vi "Hand_Store_rach.vi"() -> ()   [LabVIEW 2016]
doc: "自动采集图线程序。\n\n1. 命名只需要给出文件夹目录，base name 可以不写，否则将以 path/base-name1_1.tif，path/base-name1.5_2.tif。后面的 _2 , _1 只有 frames 大于1 才会添加。\n2. start 可以比 end大，自动递减，否则递增。\n3. one pass 表示只以 step 间隔从 start 到 end，选中 auto reverse 可以自动从 end 返回到 start，并在 基名（base name）前 加 bg_。注意 start 减 end 结果除以 step 应是整数。\n4. 每次采集完后需要点击 paused 转到 Continue，继续下一个数据的采集。\n5. force stop 可以强制退出（paused 状态下方可）。\n\n——冉成 2018.09.14"
uses:
  SUBVI/Global_Variates.vi
panel:
  in  "w2":i32=2048 min=0 max=2048 step=1
  in  "w1":i32 min=0 max=2048 step=1
  in  "h2":i32=2048 min=0 max=2048 step=1
  in  "h1":i32 min=0 max=2048 step=1
  out "cam_status":bool
  in  "auto convert2tiff":bool=TRUE caption="Blank Button"
  in  "Force Stop":bool
  out "DCAM Version":string
  out "Lib Version":string
  in  "Set":dbl=0.5
  out "Actual":dbl
  out "Frames Recorded":i32
  out "Display":T1(plugin-control)
  in  "Frames":i32=1
  in  "Parameter":u32(ring)=2049184 items=["SENSOR MODE"=4212128, "CCD MODE"=4212384, "READOUT MODE"=4211872, "ACTIVE VIEW INDEX"=4343136, "BITS PER CHANNEL"=4342976, "IMAGE PIXEL TYPE"=4343296, "BINNING"=4215968, "EXPOSURE TIME"=2049184, "CONTRAST GAIN"=3163312, "CONTRAST OFFSET"=3163328, "LIGHT MODE"=2114720, "SENSITIVITY"=2114992, "PHOTON IMAGING MODE"=2115200, "HIGH DYNAMIC RANGE MODE"=3163360, "WHITE BALANCE"=3163568, "TEMPERATURE"=2115232, "TEMPERATURE TARGET"=2115264, "SENSOR COOLER FAN"=2115296, "LINEBUNDLE HEIGHT"=4212192, "MECHANICAL SHUTTER"=2115488, "BACK FOCUS POSITION"=8422304, "TRIGGER CONNECTOR"=1066432, "TRIGGER SOURCE"=1066144, "OUTPUT TRIGGER SOURCE"=1852576, "TRIGGER GLOBAL EXPOSURE"=2049680, "FIRST TRIGGER BEHAVIOR"=2049696, "CHANNEL SYNC"=1852352, "READOUT DIRECTION"=4211904, "PRE HSYNC COUNT"=1852704, "INTERNAL LINE SPEED"=4226000, "INTERNAL LINE INTERVAL"=4226016]
  in  "Continue":bool
  in  "Auto Reverse":bool
  out "Current":dbl
  in  "Base Name":string
  in  "Folder Path":path
  in  "Step":dbl min=0.0 max=14.0 step=0.1
  in  "End":dbl min=0.0 max=14.0
  in  "Start":dbl min=0.0 max=14.0
  # "裁剪图片"
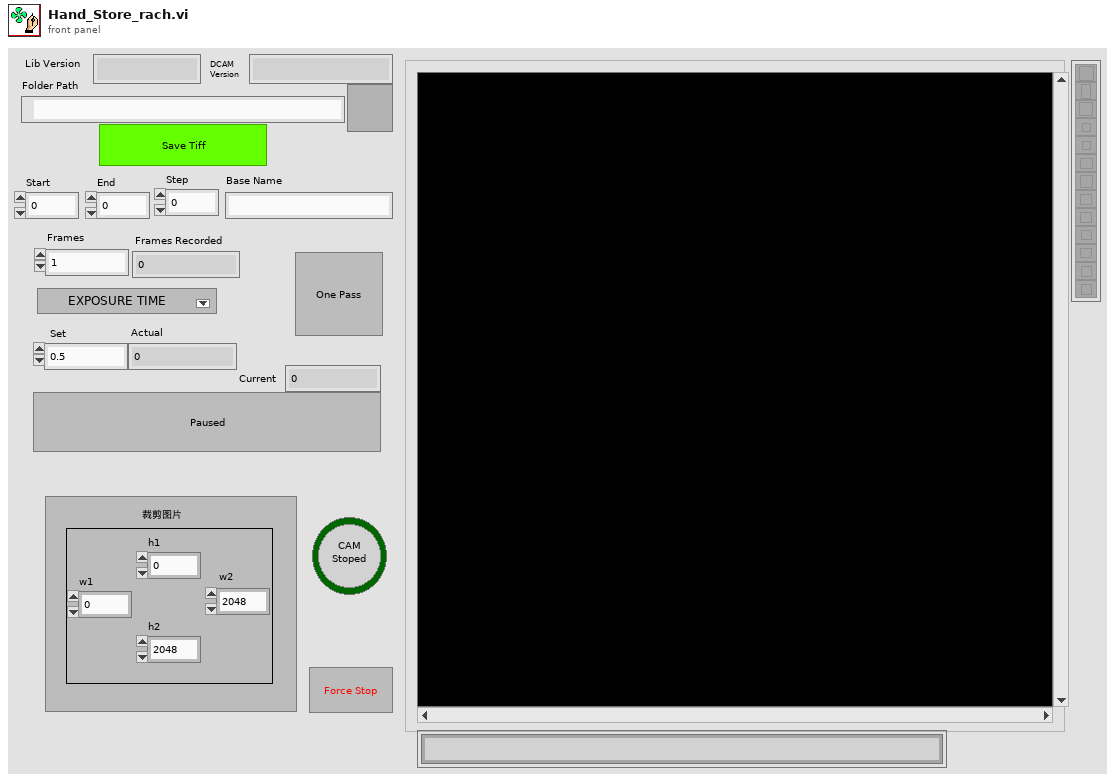
[diagram p1: front panel]
types:
  T1 = typedef "IMAQ Image.ctl" = refnum<image>
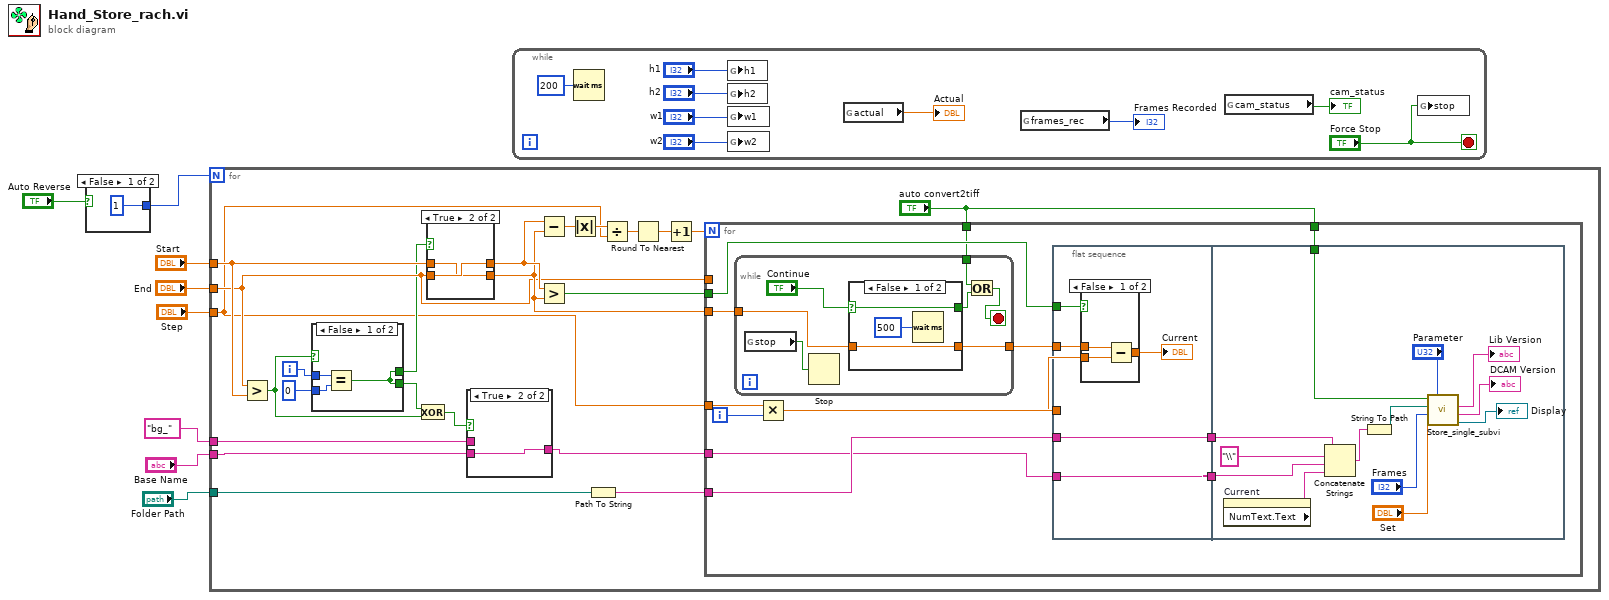
[diagram p0: block diagram]
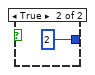
[diagram p2: hidden frame]
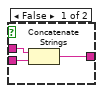
[diagram p3: hidden frame]
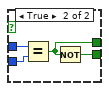
[diagram p4: hidden frame]
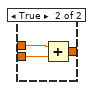
[diagram p6: hidden frame]
diagram:
  n1 = case shown="False" "Auto Reverse" {
    tunnel: [1 2] -> w1
    frame False {
    }
    frame True {
    }
  }
  n2 = for {
    N: w1 -> [_]
    tunnel: "End" -> [w22]
    tunnel: "Start" -> [w23]
    tunnel: "Step" -> [w12]
    tunnel: "Folder Path" -> [w27]
    tunnel: "Base Name" -> [w14]
    tunnel: "bg_" ("string") -> [w16]
    i -> [w26]
    n3 = Greater?(x=w22, y=w23) -> (0:w19:bool)
    n4 = case shown="False" w19 {
      tunnel: w26 -> [w40 w44]
      tunnel: 0 ("y") -> [w39 w43]
      tunnel: [w38 w41] -> w18
      tunnel: [w38 w42] -> w17
      frame False {
        n5 = Equal?(x=w40, y=w39) -> (x = y?=w38:bool)
      }
      frame True {
        n6 = Equal?(x=w44, y=w43) -> (x = y?=w41:bool)
        n7 = Not(x=w41) -> (.not. x?=w42:bool)
      }
    }
    n8 = Exclusive Or(1:w19, 2:w17) -> (0:w20:bool)
    n9 = case shown="True" w18 {
      tunnel: w22 -> [w46 w48]
      tunnel: w23 -> [w45 w47]
      tunnel: [w45 w48] -> w29
      tunnel: [w46 w47] -> w28
      frame False {
      }
      frame True {
      }
    }
    n10 = case shown="True" w20 {
      tunnel: [w36 w37] -> w15
      tunnel: w14 -> [w35 w37]
      tunnel: w16 -> [w34 _]
      frame False {
        n11 = Concatenate Strings(w34, w35) -> (w36:string)
      }
      frame True {
      }
    }
    n12 = Subtract(x=w29, y=w28) -> (x-y=w32:dbl)
    n13 = Greater?(x=w29, y=w28) -> (0:w30:bool)
    n14 = Absolute Value(x=w32) -> (abs(x)=w31:dbl)
    n15 = Path To String(path=w27) -> (string=w13:string)
    n16 = Divide(x=w31, y=w12) -> (x/y=w33:dbl)
    n17 = Round To Nearest(number=w33) -> (nearest integer value=w24:dbl)
    n18 = Increment(x=w24) -> (x+1=w25:dbl)
    n19 = for {
      N: w25 -> [_]
      tunnel: w12 -> [w59]
      tunnel: w28 -> [w58]
      tunnel: w30 -> [w55]
      tunnel: w22 -> [_]
      tunnel: w13 -> [w54]
      tunnel: w15 -> [w52]
      tunnel: "auto convert2tiff" -> [w50]
      tunnel: "auto convert2tiff" -> [w49]
      i -> [w60]
      n20 = while {
        tunnel: w58 -> [w92]
        tunnel: [w91] -> w57
        tunnel: w49 -> [w87]
        stop <- w88 stop-if-true
        n21 = global read "Global_Variates.vi" "stop"() -> (w86:bool)
        n22 = Stop(stop? (T)=w86) -> ()
        n23 = case shown="False" "Continue" {
          selector: "Continue" -> [w95 w97]
          tunnel: [w95 w97] -> w89
          tunnel: w92 -> [w93 w96]
          tunnel: [w93 w96] -> w91
          frame False {
            n24 = Wait (ms)(milliseconds to wait=u32 500) -> ()  [unwired: 1 out]
          }
          frame True {
          }
        }
        n25 = Or(x=w87, y=w89) -> (x .or. y?=w88:bool)
      }
      n26 = Multiply(x=w59, y=w60) -> (x*y=w56:dbl)
      n27 = flat-sequence {
        tunnel: w57 -> [w66]
        tunnel: w56 -> [w61]
        tunnel: w55 -> [w64]
        tunnel: w54 -> [w63]
        tunnel: [w63] -> w53
        tunnel: w52 -> [w62]
        tunnel: [w62] -> w51
        tunnel: w53 -> [w77]
        tunnel: w51 -> [w76]
        tunnel: w50 -> [w74]
        frame #0 {
          n28 = case shown="False" w64 {
            tunnel: w61 -> [w67 w72]
            tunnel: w66 -> [w68 w71]
            tunnel: [w69 w70] -> w65
            frame False {
              n29 = Subtract(x=w68, y=w67) -> (x-y=w69:dbl)
            }
            frame True {
              n30 = Add(x=w71, y=w72) -> (x+y=w70:dbl)
            }
          }
          "Current" <- w65
        }
        frame #1 {
          n31 = property on="Current" class="DigNum (strict)"() -> ("NumText.Text"=w73:string)  [unwired: 2 in, 2 out]
          n32 = Concatenate Strings(w77, "\\" ("string"), w76, w73) -> (w83:string)
          n33 = String To Path(string=w83) -> (path=w84:path)
          n34 = call "Store_single_subvi.vi"("Parameter"="Parameter", "Set"="Set", "Frames"="Frames", "File"=w84, "save"=w74) -> ("Display"=→"Display":T1, "DCAM Version"=→"DCAM Version":string, "Library Version"=→"Lib Version":string)
        }
      }
    }
  }
  n35 = while {
    stop <- "Force Stop" stop-if-true
    n36 = Wait (ms)(milliseconds to wait=u32 200) -> ()  [unwired: 1 out]
    n37 = global write "Global_Variates.vi" "h1"("h1") -> ()
    n38 = global write "Global_Variates.vi" "h2"("h2") -> ()
    n39 = global write "Global_Variates.vi" "w1"("w1") -> ()
    n40 = global write "Global_Variates.vi" "w2"("w2") -> ()
    n41 = global read "Global_Variates.vi" "actual"() -> (→"Actual":dbl)
    n42 = global read "Global_Variates.vi" "frames_rec"() -> (→"Frames Recorded":i32)
    n43 = global read "Global_Variates.vi" "cam_status"() -> (→"cam_status":bool)
    n44 = global write "Global_Variates.vi" "stop"("Force Stop") -> ()
  }
